vi "Main.vi"() -> ()   [LabVIEW 2017, in "WebServiceImporter.lvlib" / "Main Panel.lvlib" / "Finish.lvlib"]
uses:
  <vilib>/Platform/WebService/Main Panel/Pages/Finish/Finish.lvlib
  <vilib>/Platform/WebService/Main Panel/Pages/Finish/Data Type/Enable Disable.ctl
  <vilib>/Platform/WebService/Global/Const Strings.vi
  <vilib>/Platform/WebService/Main Panel/Pages/Finish/Events/Events.lvlib
  <vilib>/Platform/WebService/Main Panel/Main Panel.lvlib
  <vilib>/Platform/WebService/WebServiceImporter.lvlib
  <vilib>/Platform/WebService/VI Generator/VI Generator.lvlib
  <vilib>/Platform/WebService/Error Handling/Error Handling.lvlib
panel:
  in  "Panel":enum32{"Interface Frame", "Hidden Controls"}(tab)
  in  "View report":bool
  in  "Open imported project library":bool
  out "Status":string
  # "Completed"
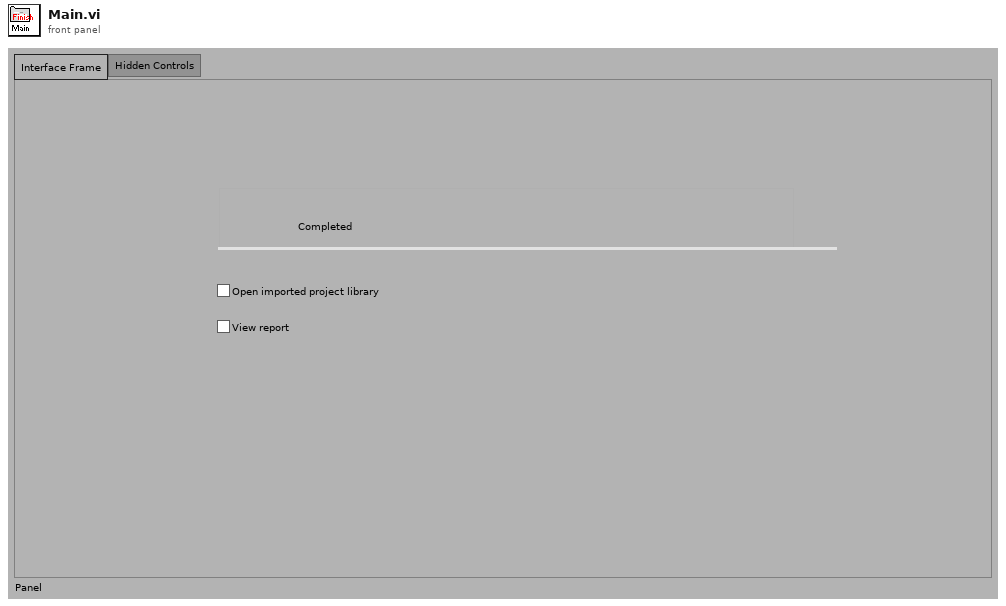
[diagram p1: front panel]
types:
  T1 = typedef "WebServiceImporter.lvlib/Main Panel.lvlib/Finish.lvlib/Enable Disable.ctl" = enum8{"Enabled", "Disabled", "Disabled and Grayed Out"}
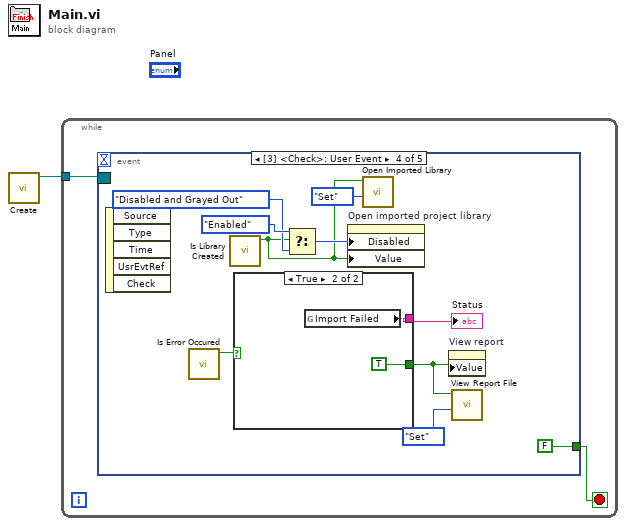
[diagram p0: block diagram]
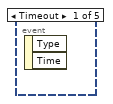
[diagram p2: hidden frame]
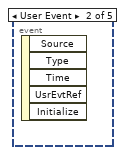
[diagram p3: hidden frame]
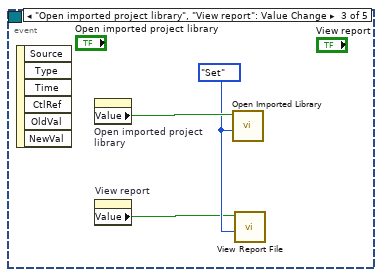
[diagram p4: hidden frame]
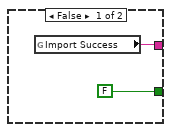
[diagram p5: hidden frame]
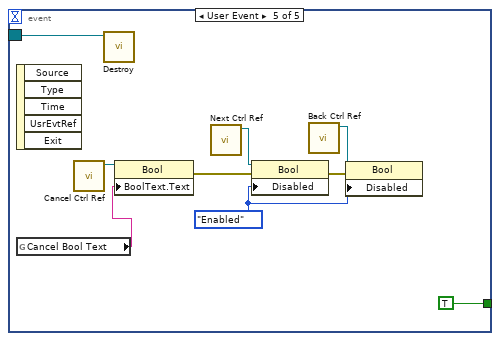
[diagram p6: hidden frame]
diagram:
  n1 = call <vilib>:"Create.vi"() -> ("Event Registration Refnum"=w1:refnum<event-registration>)  [unwired: 10 in, 1 out]
  n2 = while {
    tunnel: w1 -> [w3]
    stop <- w2 stop-if-true
    n3 = event shown="[3] <Check>: User Event" {
      selector: w3 -> [_ _ _ _ w29]
      dyn-events: _ -> [_ _ _ _ _]
      timeout: _ -> [_ _ _ _ _]
      tunnel: [_ _ _ FALSE TRUE] -> w2
      event Timeout {
        n4 = event-data() -> ()  [unwired: 1 in, 2 out]
      }
      event User Event {
        n5 = event-data() -> ()  [unwired: 1 in, 5 out]
      }
      event "Open imported project library", "View report": Value Change {
        w5 = enum16{"Get", "Set"}."Set" ("Operation")
        n6 = event-data() -> ()  [unwired: 1 in, 6 out]
        n7 = property on="Open imported project library" class="Bool (strict)"() -> ("Value"=w6:bool)  [unwired: 2 in, 2 out]
        n8 = property on="View report" class="Bool (strict)"() -> ("Value"=w4:bool)  [unwired: 2 in, 2 out]
        n9 = call <vilib>:"Open Imported Library.vi"("Operation"=w5, "Boolean"=w6) -> ()  [unwired: 8 in, 2 out]
        n10 = call <vilib>:"View Report File.vi"("Operation"=w5, "Boolean"=w4) -> ()  [unwired: 8 in, 2 out]
      }
      event User Event {
        n11 = event-data() -> ()  [unwired: 1 in, 5 out]
        n12 = call <vilib>:"Is Error Occured.vi"() -> ("Error Occured?  2"=w16:bool)  [unwired: 10 in, 1 out]
        n13 = call <vilib>:"Is Library Created.vi"() -> ("Created? 2"=w8:bool)  [unwired: 10 in, 1 out]
        n14 = case shown="True" w16 {
          tunnel: [w18 w20] -> w15
          tunnel: [FALSE TRUE] -> w10
          frame False {
            n15 = global read "Const Strings.vi" "Import Success"() -> (w18:string)
          }
          frame True {
            n16 = global read "Const Strings.vi" "Import Failed"() -> (w20:string)
          }
        }
        "Status" <- w15
        n17 = Select(t=Enable_Disable."Enabled" ("Disabled"), s=w8, f=Enable_Disable."Disabled and Grayed Out" ("Disabled")) -> (s? t:f=w11:T1)
        n18 = property on="Open imported project library" class="Bool (strict)"("Disabled"=w11, "Value"=w8) -> ()  [unwired: 2 in, 2 out]
        n19 = call <vilib>:"Open Imported Library.vi"("Operation"=enum16{"Get", "Set"}."Set", "Boolean"=w8) -> ()  [unwired: 8 in, 2 out]
        n20 = property on="View report" class="Bool (strict)"("Value"=w10) -> ()  [unwired: 2 in, 2 out]
        n21 = call <vilib>:"View Report File.vi"("Operation"=enum16{"Get", "Set"}."Set", "Boolean"=w10) -> ()  [unwired: 8 in, 2 out]
      }
      event User Event {
        w23 = Enable_Disable."Enabled" ("Disabled")
        n22 = event-data() -> ()  [unwired: 1 in, 5 out]
        n23 = global read "Const Strings.vi" "Cancel Bool Text"() -> (w21:string)
        n24 = call <vilib>:"Cancel Ctrl Ref.vi"() -> ("Ctl Refnum (out)"=w27:refnum<vi>)  [unwired: 11 in]
        n25 = call <vilib>:"Destroy.vi"("Event Registration Refnum"=w29) -> ()  [unwired: 10 in, 1 out]
        n26 = property class="Bool"(reference=w27, "BoolText.Text"=w21) -> (error out=w22:errorcluster)  [unwired: 1 in, 1 out]
        n27 = call <vilib>:"Next Ctrl Ref.vi"() -> ("Ctl Refnum (out)"=w26:refnum<vi>)  [unwired: 10 in, 1 out]
        n28 = property class="Bool"(reference=w26, error in=w22, "Disabled"=w23) -> (error out=w24:errorcluster)  [unwired: 1 out]
        n29 = call <vilib>:"Back Ctrl Ref.vi"() -> ("Ctl Refnum (out)"=w25:refnum<vi>)  [unwired: 10 in, 1 out]
        n30 = property class="Bool"(reference=w25, error in=w24, "Disabled"=w23) -> ()  [unwired: 2 out]
      }
    }
  }
